vi "niRFUtil RFHS Channelizer CreateChannelizer CSG.vi"(0 "Channelizer Spec":T3={"freq in Hz"=TRUE, "Filter Type Hint"=enum."FFT (LTE)", "Hint Value"=0.5, "Channels"=[]} {"Channels"."Flags" items=["None"=0, "Force Fractional"=1, "Use Multistage"=2, "Use Pretrigger Data "=256, "Frequency Shift Only"=4]; "Channels"."fs" format="%#_8p"; "Channels"."fc" format="%#_6p"; "Channels"."stopBW" format="%#_6p"; "Channels"."passBW" format="%#_6p"; "Hint Value" format="%#_8p"}, 1 "Type":T1, 2 "Benchmark Task":T8, 3 "Replace Filter Data":bool, 5 "fs [Hz]":dbl=1000000000.0 format="%#_6p", 7 "Mode":T2, 9 "Buffer Size (s)":dbl=0.003 format="%#_6p", 11 "error in (no error)":errorcluster, 13 "User Filter Spec":T7) -> (4 "Channelizer Ref":refnum<data-value>, 15 "error out":errorcluster)   [LabVIEW 2015, in "niRFUtil.lvlib"]
uses:
  niRFUtil.lvlib
  Utilities/Benchmark/niRFUtil RFHS Benchmark Task.ctl
  Utilities/niRFUtil RFHS Util User Filter Specification.ctl
  Includes/niRFUtil RFHS Channelizer ChannelSpecification.ctl
  Includes/niRFUtil RFHS Channelizer FilterTypeHint.ctl
  Includes/niRFUtil RFHS Channelizer ChannelSpecificationBase.ctl
  Includes/niRFUtil RFHS Channelizer ChannelFlags.ctl
  Includes/niRFUtil RFHS Channelizer ChannelizerBufferingMode.ctl
  Includes/niRFUtil RFHS Channelizer ChannelizerInfo CSG.ctl
  Includes/niRFUtil RFHS Channelizer FilterRef.ctl
  Utilities/Data FIFO/niRFUtil RFHS FIFO Reference.ctl
  Utilities/Data FIFO/niRFUtil RFHS FIFO.ctl
  Includes/niRFUtil RFHS Channelizer ChannelizerType.ctl
  Includes/niRFUtil RFHS Channelizer ChannelizerFlags.ctl
panel:
  in  "Inital Phase":dbl
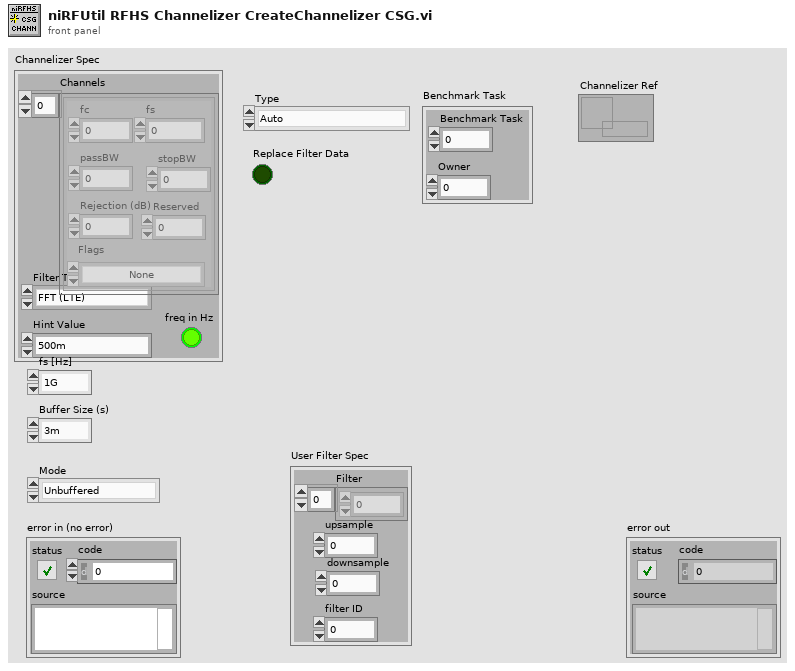
[diagram p1: front panel]
types:
  T1 = typedef "niRFUtil.lvlib/niRFUtil RFHS Channelizer ChannelizerType.ctl" = enum32{"Auto", "Frequency Shift Only", "Resampler Only"}
  T2 = typedef "niRFUtil.lvlib/niRFUtil RFHS Channelizer ChannelizerBufferingMode.ctl" = enum32{"Unbuffered", "Finite", "Continuous"}
  T3 = typedef "niRFUtil.lvlib/niRFUtil RFHS Channelizer ChannelSpecification.ctl" = cluster{"freq in Hz":bool, "Filter Type Hint":T4, "Hint Value":dbl, "Channels":T5[]}
  T4 = typedef "niRFUtil.lvlib/niRFUtil RFHS Channelizer FilterTypeHint.ctl" = enum16{"Auto", "FFT (LTE)", "FFT (WiFi)", "FFT (custom)"}
  T5 = typedef "niRFUtil.lvlib/niRFUtil RFHS Channelizer ChannelSpecificationBase.ctl" = cluster{"fc":dbl, "fs":dbl, "passBW":dbl, "stopBW":dbl, "Rejection (dB)":dbl, "Flags":T6, "Reserved":i32}
  T6 = typedef "niRFUtil.lvlib/niRFUtil RFHS Channelizer ChannelFlags.ctl" = u32
  T7 = typedef "niRFUtil.lvlib/niRFUtil RFHS Util User Filter Specification.ctl" = cluster{"Filter":dbl[], "upsample":i32, "downsample":i32, "filter ID":i32}
  T8 = typedef "niRFUtil.lvlib/niRFUtil RFHS Benchmark Task.ctl" = cluster{"Benchmark Task":u64, "Owner":u32}
  T9 = typedef "niRFUtil.lvlib/niRFUtil RFHS Channelizer ChannelizerInfo CSG.ctl" = cluster{"Filter LVRef":T10, "Mode":T2, "History":csg[], "Buffer":csg[], "FIFO":T11, "History Len":u32, "Float Cache":csg[], "Double Cache":cdb[], "Type":T1, "Resample Phase":dbl, "fft1Descriptors":u64[], "fft2Descriptors":u64[], "FFT tBuf":csg[], "guardBandLen":i32, "FFT History":csg[], "FFT History Len":u32, "FFTInitDone":u32, "FFT Filter LVRefs":T10[], "FFT fc Offs":u32[], "fft2Sizes":u32[], "BufferW":u32[], "BufferR":u32[], "Buff Off":u32[], "Phase0 (fshift)":dbl[], "Phase (fshift)":dbl[], "fs phase step":dbl[], "Resample Step":dbl, "Flags":T13, "Reset Cnt":i64, "Filter Pass":u32, "Stages":variant[]}
  T10 = typedef "niRFUtil.lvlib/niRFUtil RFHS Channelizer FilterRef.ctl" = cluster{"Ref":u64, "GUID":u64, "Upsample":i32, "Downsample":i32, "Size":i32, "Num Taps":i32}
  T11 = typedef "niRFUtil.lvlib/niRFUtil RFHS FIFO Reference.ctl" = cluster{"Read Lock":refnum<data-value>, "Info":T12, "Write Lock":refnum<data-value>}
  T12 = typedef "niRFUtil.lvlib/niRFUtil RFHS FIFO.ctl" = cluster{"ID":u64, "Length":u32}
  T13 = typedef "niRFUtil.lvlib/niRFUtil RFHS Channelizer ChannelizerFlags.ctl" = u32
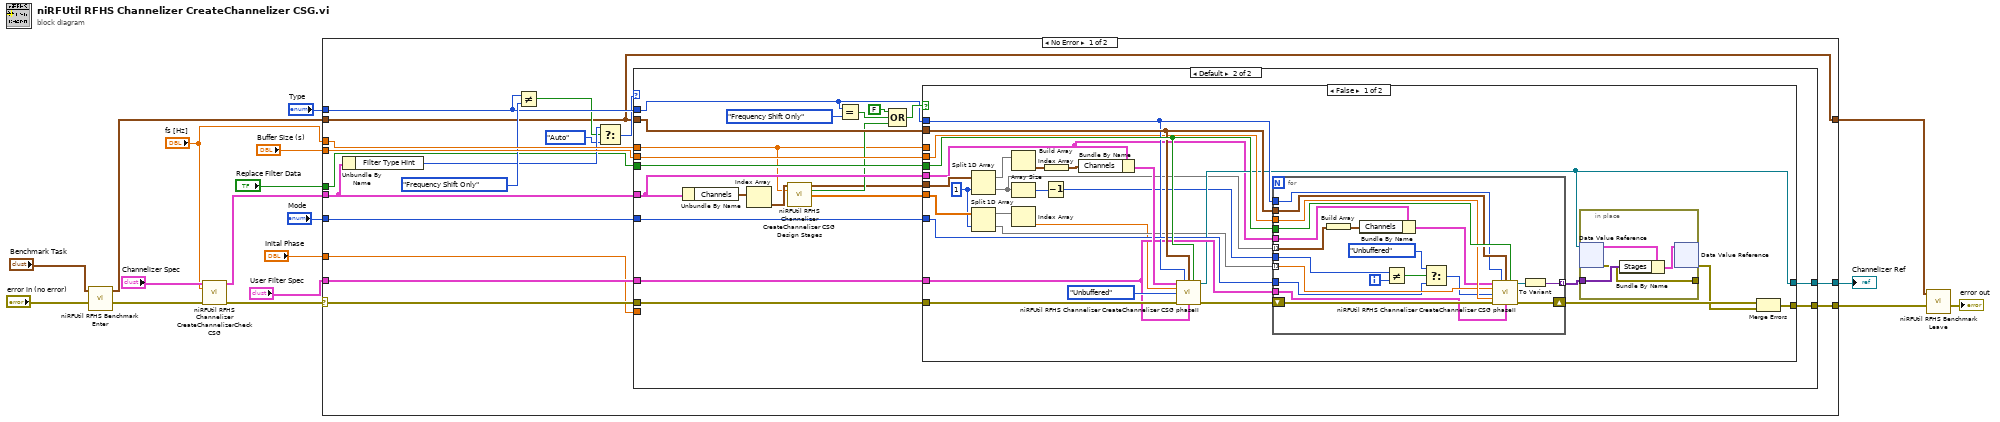
[diagram p0: block diagram]
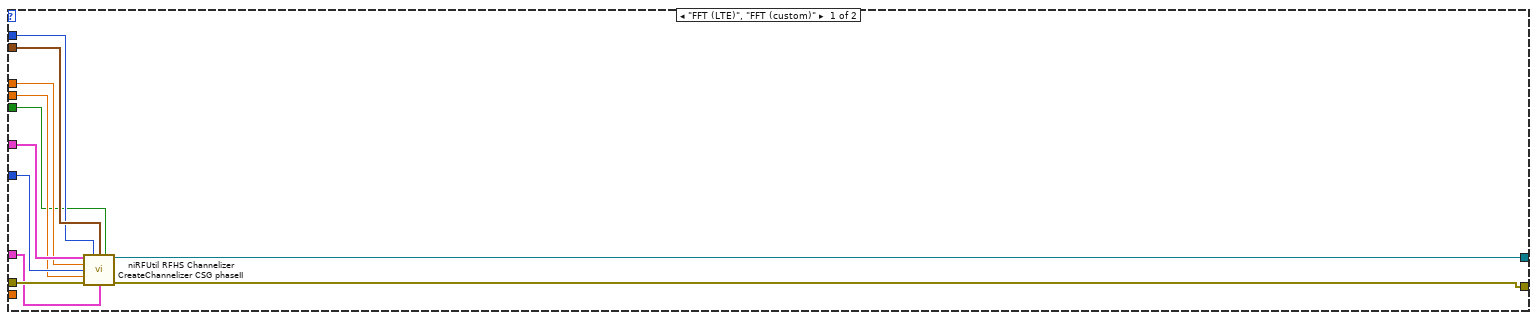
[diagram p2: hidden frame]
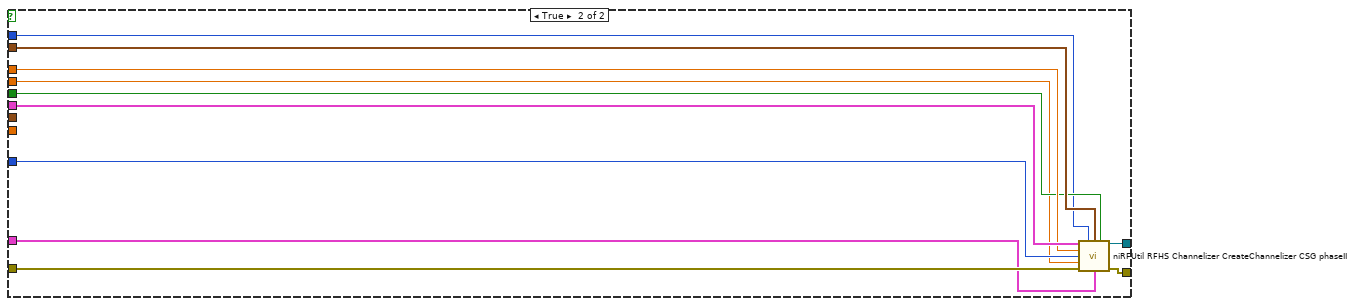
[diagram p3: hidden frame]
diagram:
  n1 = call "niRFUtil RFHS Benchmark Enter.vi"("error in (no error)"="error in (no error)", "Benchmark Task (Parent)"="Benchmark Task") -> ("error out"=w5:errorcluster, "Benchmark Task (Self)"=w7:T8)  [unwired: 8 in]
  n2 = call "niRFUtil RFHS Channelizer CreateChannelizerCheck CSG.vi"("Channel Spec"="Channelizer Spec", "fs [Hz]"="fs [Hz]", "error in (no error)"=w5) -> ("Channel Spec (out)"=w1:T3, "error out"=w4:errorcluster)  [unwired: 11 in]
  n3 = case shown="No Error" w4 {
    selector: w4 -> [w35 w131]
    tunnel: [w19 w131] -> w17
    tunnel: w1 -> [w22 _]
    tunnel: "fs [Hz]" -> [w32 _]
    tunnel: "User Filter Spec" -> [w34 _]
    tunnel: "Mode" -> [w31 _]
    tunnel: "Type" -> [w28 _]
    tunnel: w7 -> [w20 w130]
    tunnel: [w21 _] -> w11
    tunnel: "Buffer Size (s)" -> [w33 _]
    tunnel: "Inital Phase" -> [w24 _]
    tunnel: "Replace Filter Data" -> [w26 _]
    tunnel: [w20 w130] -> w6
    frame No Error {
      n4 = Unbundle By Name(w22) -> ("Filter Type Hint"=w29:T4)
      n5 = Not Equal?(x=w28, y=niRFUtil_RFHS_Channelizer_ChannelizerType."Frequency Shift Only") -> (x != y?=w27:bool)
      n6 = Select(t=w29, s=w27, f=niRFUtil_RFHS_Channelizer_FilterTypeHint."Auto") -> (s? t:f=w23:T4)
      n7 = case shown="Default" w23 {
        tunnel: w35 -> [w42 w56]
        tunnel: w34 -> [w38 w54]
        tunnel: [w41 w55] -> w19
        tunnel: w33 -> [w39 w57]
        tunnel: w32 -> [w45 w47]
        tunnel: w22 -> [w46 w62]
        tunnel: w31 -> [w40 w58]
        tunnel: w20 -> [w43 w61]
        tunnel: w28 -> [w37 w59]
        tunnel: w26 -> [w36 w60]
        tunnel: w24 -> [_ _]
        tunnel: [w44 w53] -> w21
        frame "FFT (LTE)", "FFT (custom)" {
          n8 = call "niRFUtil RFHS Channelizer CreateChannelizer CSG phaseII.vi"("Channelizer Spec"=w46, "Type"=w37, "Benchmark Task"=w43, "Replace Filter Data"=w36, "fs [Hz]"=w45, "Mode"=w40, "Buffer Size (s)"=w39, "error in (no error)"=w42, "User Filter Spec"=w38) -> ("Channelizer Ref"=w44:refnum<data-value>, "error out"=w41:errorcluster)  [unwired: 5 in]
        }
        frame Default {
          n9 = Unbundle By Name(w62) -> ("Channels"=w65:T5[])
          n10 = Index Array(array=w65) -> (element=w51:T5)  [unwired: 1 in]
          n11 = call "niRFUtil RFHS Channelizer CreateChannelizer CSG Design Stages.vi"("Channel Spec"=w51, "fs"=w47) -> ("Stages"=w49:T5[], "Single Stage"=w50:bool, "fs List"=w48:dbl[])  [unwired: 11 in]
          n12 = Equal?(x=w59, y=niRFUtil_RFHS_Channelizer_ChannelizerType."Frequency Shift Only") -> (x = y?=w64:bool)
          n13 = Compound Arithmetic op=OR(FALSE ("value"), w64, w50) -> (w63:bool)
          n14 = case shown="False" w63 {
            tunnel: w62 -> [w78 w129]
            tunnel: w47 -> [_ w128]
            tunnel: w61 -> [w89 w127]
            tunnel: w60 -> [w90 w126]
            tunnel: w59 -> [w86 w125]
            tunnel: w58 -> [w87 w124]
            tunnel: w57 -> [w84 w123]
            tunnel: w56 -> [w94 w122]
            tunnel: [w82 w121] -> w55
            tunnel: w54 -> [w85 w120]
            tunnel: [w83 w119] -> w53
            tunnel: w49 -> [w81 _]
            tunnel: w48 -> [w76 _]
            frame False {
              w74 = 1 ("index")
              n15 = Split 1D Array(array=w81, index=w74) -> (first subarray=w80:T5[], second subarray=w69:T5[])
              n16 = Split 1D Array(array=w76, index=w74) -> (first subarray=w73:dbl[], second subarray=w75:dbl[])
              n17 = Index Array(array=w80) -> (element=w79:T5)  [unwired: 1 in]
              n18 = Array Size(array=w69) -> (size(s)=w68:i32)
              n19 = Index Array(array=w73) -> (element=w72:dbl)  [unwired: 1 in]
              n20 = Decrement(x=w68) -> (x-1=w67:i32)
              n21 = Build Array(w79) -> (w93:T5[])
              n22 = Bundle By Name(cluster=w78, "Channels"=w93) -> (w92:T3)
              n23 = call "niRFUtil RFHS Channelizer CreateChannelizer CSG phaseII.vi"("Channelizer Spec"=w92, "Type"=w86, "Benchmark Task"=w89, "Replace Filter Data"=w90, "fs [Hz]"=w72, "Mode"=niRFUtil_RFHS_Channelizer_ChannelizerBufferingMode."Unbuffered", "error in (no error)"=w94, "User Filter Spec"=w85) -> ("Channelizer Ref"=w83:refnum<data-value>, "error out"=w91:errorcluster)  [unwired: 6 in]
              n24 = for {
                tunnel: w90 -> [w113]
                tunnel: w89 -> [w112]
                tunnel: w87 -> [w96]
                tunnel: w86 -> [w111]
                tunnel: w85 -> [w110]
                tunnel: w84 -> [w109]
                tunnel: w78 -> [w107]
                tunnel: w69 -> [w106] mode=indexing
                tunnel: [w103] -> w77 mode=indexing
                tunnel: w75 -> [w102] mode=indexing
                shift-right: [w108] -> w71
                shift-left: w91 -> [w114]
                tunnel: w67 -> [w100]
                i -> [w99]
                n25 = Build Array(w106) -> (w105:T5[])
                n26 = Bundle By Name(cluster=w107, "Channels"=w105) -> (w101:T3)
                n27 = Not Equal?(x=w100, y=w99) -> (x != y?=w98:bool)
                n28 = Select(t=niRFUtil_RFHS_Channelizer_ChannelizerBufferingMode."Unbuffered" ("Mode"), s=w98, f=w96) -> (s? t:f=w95:T2)
                n29 = call "niRFUtil RFHS Channelizer CreateChannelizer CSG phaseII.vi"("Channelizer Spec"=w101, "Type"=w111, "Benchmark Task"=w112, "Replace Filter Data"=w113, "fs [Hz]"=w102, "Mode"=w95, "Buffer Size (s)"=w109, "error in (no error)"=w114, "User Filter Spec"=w110) -> ("Channelizer Ref"=w104:refnum<data-value>, "error out"=w108:errorcluster)  [unwired: 5 in]
                n30 = To Variant(anything=w104) -> (Variant=w103:variant)
              }
              n31 = in-place {
                in-place-border: w77 -> [w116]
                in-place-border: [w115] -> _
                n32 = in-place-dvr #1(w83) -> (w118:T9, w115:errorcluster)
                n33 = Bundle By Name(cluster=w118, "Stages"=w116) -> (w117:T9)
                n34 = in-place-dvr #1(w117) -> (w70:errorcluster)  [unwired: 1 out]
              }
              n35 = Merge Errors(w71, w70) -> (w82:errorcluster)
            }
            frame True {
              n36 = call "niRFUtil RFHS Channelizer CreateChannelizer CSG phaseII.vi"("Channelizer Spec"=w129, "Type"=w125, "Benchmark Task"=w127, "Replace Filter Data"=w126, "fs [Hz]"=w128, "Mode"=w124, "Buffer Size (s)"=w123, "error in (no error)"=w122, "User Filter Spec"=w120) -> ("Channelizer Ref"=w119:refnum<data-value>, "error out"=w121:errorcluster)  [unwired: 5 in]
            }
          }
        }
      }
    }
    frame Error {
    }
  }
  "Channelizer Ref" <- w11
  n37 = call "niRFUtil RFHS Benchmark Leave.vi"("error in (no error)"=w17, "Benchmark Task Self"=w6) -> ("error out"=→"error out":errorcluster)  [unwired: 8 in, 1 out]
